vi "magnet_controller.vi"(1 "Arguments":string, 2 "Command":T1(ring)=enum."Hold", 3 "Direction":enum16{"X", "Y", "Z"}(ring)=enum."Y") -> (0 "Response":string)   [LabVIEW 2010]
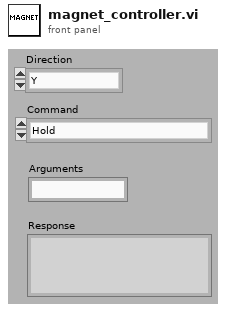
[diagram p1: front panel]
types:
  T1 = enum16{"Read State", "Hold", "Ramp to Set", "Ramp to Zero", "Read Switch Heater", "Switch Heater On", "Switch Heater Off", "Read Voltage", "Read Current", "Read Field", "Read Persistent Field", "Read Target Field", "Set Target Field", "Read Ramp Rate", "Set Ramp Rate"}
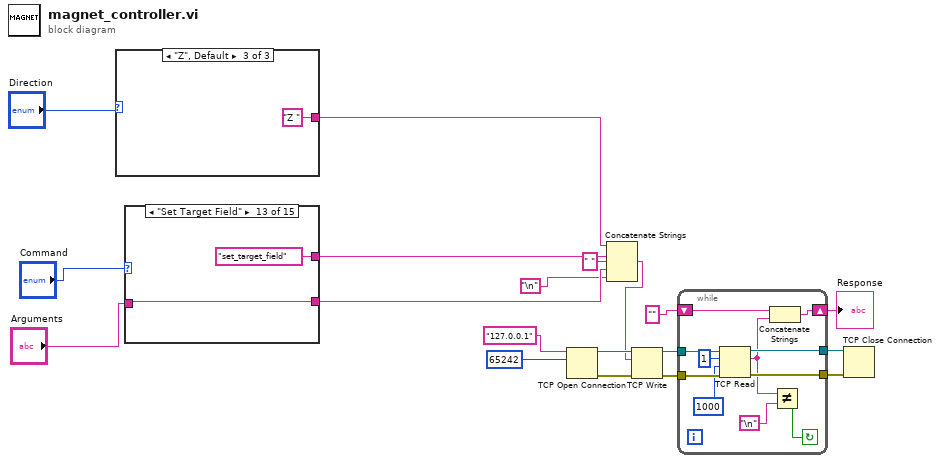
[diagram p0: block diagram]
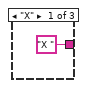
[diagram p2: hidden frame]
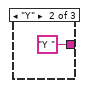
[diagram p3: hidden frame]
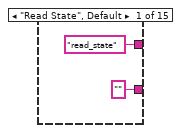
[diagram p4: hidden frame]
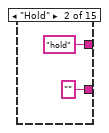
[diagram p5: hidden frame]
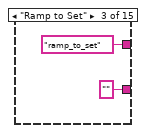
[diagram p6: hidden frame]
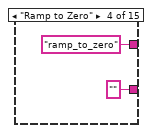
[diagram p7: hidden frame]
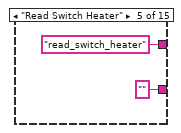
[diagram p8: hidden frame]
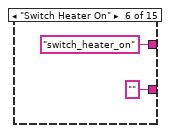
[diagram p9: hidden frame]
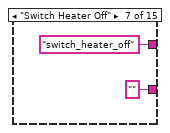
[diagram p10: hidden frame]
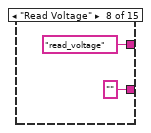
[diagram p11: hidden frame]
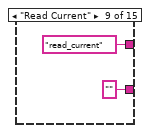
[diagram p12: hidden frame]
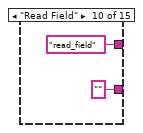
[diagram p13: hidden frame]
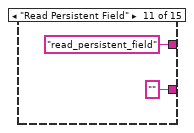
[diagram p14: hidden frame]
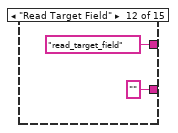
[diagram p15: hidden frame]
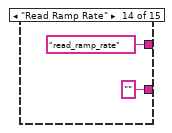
[diagram p16: hidden frame]
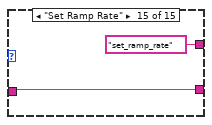
[diagram p17: hidden frame]
diagram:
  n1 = case shown="\"Z\", Default" "Direction" {
    tunnel: ["X " ("string") "Y " ("string") "Z " ("string")] -> w1
    frame "X" {
    }
    frame "Y" {
    }
    frame "Z", Default {
    }
  }
  n2 = case shown="\"Set Target Field\"" "Command" {
    tunnel: ["read_state" ("data in") "hold" ("data in") "ramp_to_set" ("data in") "ramp_to_zero" ("data in") "read_switch_heater" ("data in") "switch_heater_on" ("data in") "switch_heater_off" ("data in") "read_voltage" ("data in") "read_current" ("data in") "read_field" ("data in") "read_persistent_field" ("data in") "read_target_field" ("data in") "set_target_field" ("data in") "read_ramp_rate" ("data in") "set_ramp_rate" ("data in")] -> w8
    tunnel: ["" ("Arguments") "" ("Arguments") "" ("Arguments") "" ("Arguments") "" ("Arguments") "" ("Arguments") "" ("Arguments") "" ("Arguments") "" ("Arguments") "" ("Arguments") "" ("Arguments") "" ("Arguments") w47 "" ("Arguments") w51] -> w5
    tunnel: "Arguments" -> [_ _ _ _ _ _ _ _ _ _ _ _ w47 _ w51]
    frame "Read State", Default {
    }
    frame "Hold" {
    }
    frame "Ramp to Set" {
    }
    frame "Ramp to Zero" {
    }
    frame "Read Switch Heater" {
    }
    frame "Switch Heater On" {
    }
    frame "Switch Heater Off" {
    }
    frame "Read Voltage" {
    }
    frame "Read Current" {
    }
    frame "Read Field" {
    }
    frame "Read Persistent Field" {
    }
    frame "Read Target Field" {
    }
    frame "Set Target Field" {
    }
    frame "Read Ramp Rate" {
    }
    frame "Set Ramp Rate" {
    }
  }
  n3 = TCP Open Connection(address="127.0.0.1", remote port or service name=u16 65242) -> (connection ID=w17:refnum<k5>, error out=w16:errorcluster)  [unwired: 3 in]
  n4 = Concatenate Strings(w1, w8, " " ("string"), w5, "\n") -> (w9:string)
  n5 = TCP Write(connection ID=w17, data in=w9, error in (no error)=w16) -> (connection ID out=w14:refnum<k5>, error out=w15:errorcluster)  [unwired: 1 in, 1 out]
  n6 = while {
    tunnel: w15 -> [w63]
    tunnel: w14 -> [w62]
    tunnel: [w61] -> w13
    tunnel: [w60] -> w12
    shift-right: [w56] -> w10
    shift-left: "" ("string") -> [w57]
    stop <- w55 continue-if-true
    n7 = TCP Read(connection ID=w62, bytes to read=1, error in (no error)=w63, 9:1000 ("timeout ms (25000)")) -> (connection ID out=w60:refnum<k5>, data out=w54:string, error out=w61:errorcluster)  [unwired: 1 in]
    n8 = Concatenate Strings(w57, w54) -> (w56:string)
    n9 = Not Equal?(x=w54, y="\n") -> (x != y?=w55:bool)
  }
  "Response" <- w10
  n10 = TCP Close Connection(connection ID=w12, error in (no error)=w13) -> ()  [unwired: 1 in, 2 out]
